vi "Simple TCP Test.vi"() -> ()   [LabVIEW 2020, in "VectoScratch.lvlib"]
uses:
  VectoScratch.lvlib
  Vecto/Connection State.ctl
  Vecto/proto/TcpClientHello/Data.ctl
  Simple TCP Handler/Simple TCP Handler.lvclass
  C:/dev/lv 2020/lv-vecto/Vecto/TCPConnectionHandler/TCPConnectionHandler.lvclass
  C:/dev/lv 2020/lv-vecto/Vecto/TCPMessageHandler/TCPMessageHandler.lvclass
  Vecto/TCPMessaging/TCPMessaging.lvclass
  Vecto/TCPMessageService/TCPMessageAPI.lvclass
  Vecto/proto/TcpClientHello/TcpClientHello.lvlib
  Vecto/Vecto.lvlib
panel:
  out "Server Read":i32
  out "Client Read":i32
  out "Server Send":i32
  in  "Server Stop":bool
  in  "Client Stop":bool
  out "Client Send":i32
  out "Server Error":errorcluster
  out "Client Error":errorcluster
  out "Server State":T1=enum."Disconnected"
  out "Client State":T1=enum."Disconnected"
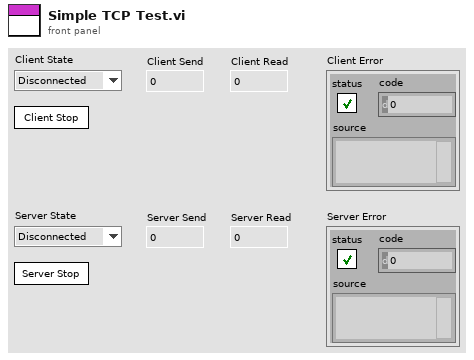
[diagram p1: front panel]
types:
  T1 = typedef "Vecto.lvlib/Connection State.ctl" = enum16{"Connected", "Disconnected"}
  T2 = typedef "TcpClientHello.lvlib/Data.ctl" = cluster{"node_id":u32, "system":string, "cluster":string, "node_name":string, "app_version":string, "config_version":string}
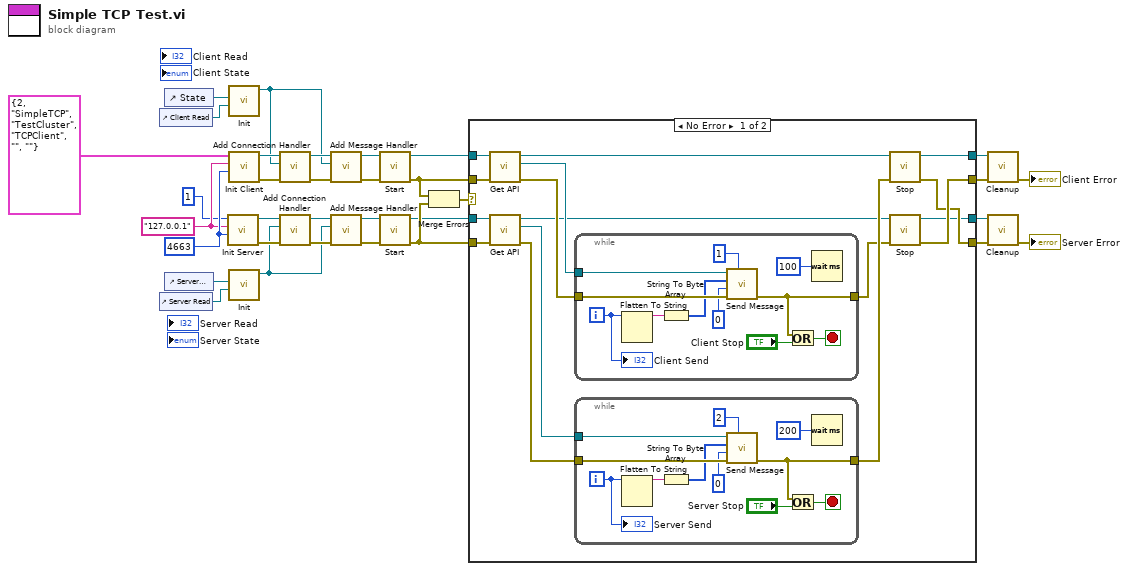
[diagram p0: block diagram]
diagram:
  w33 = u16 4663 ("Bind Port")
  w32 = "127.0.0.1" ("Bind Address")
  n1 = control-ref of="Client Read"() -> (w3:refnum<vi>)
  n2 = control-ref of="Server Read"() -> (w4:refnum<vi>)
  n3 = control-ref of="State"() -> (w30:refnum<vi>)
  n4 = control-ref of="Server State"() -> (w22:refnum<vi>)
  n5 = call "Init Server.vi"("Bind Port"=w33, "Bind Address"=w32, "Node ID"=u32 1) -> ("error out"=w16:errorcluster, "TCPMessaging out"=w17:refnum<class "TCPMessaging.lvclass">)  [unwired: 7 in]
  n6 = call "Init.vi"("Value"=w3, "State"=w30) -> ("Simple TCP Handler out"=w26:refnum<class "Simple TCP Handler.lvclass">)  [unwired: 8 in, 1 out]
  n7 = call "Init Client.vi"("Remote Port"=w33, "Remote Address"=w32, "Client Info"=T2 {"node_id"=2, "system"="SimpleTCP", "cluster"="TestCluster", "node_name"="TCPClient", "app_version"="", "config_version"=""}) -> ("error out"=w28:errorcluster, "TCPMessaging out"=w29:refnum<class "TCPMessaging.lvclass">)  [unwired: 7 in]
  n8 = call "Init.vi"("Value"=w4, "State"=w22) -> ("Simple TCP Handler out"=w2:refnum<class "Simple TCP Handler.lvclass">)  [unwired: 8 in, 1 out]
  n9 = call "Add Connection Handler.vi"("error in (no error)"=w28, "TCPConnectionHandler"=w26, "TCPMessaging in"=w29) -> ("error out"=w25:errorcluster, "TCPMessaging out"=w27:refnum<class "TCPMessaging.lvclass">)  [unwired: 7 in]
  n10 = call "Add Connection Handler.vi"("error in (no error)"=w16, "TCPConnectionHandler"=w2, "TCPMessaging in"=w17) -> ("error out"=w19:errorcluster, "TCPMessaging out"=w18:refnum<class "TCPMessaging.lvclass">)  [unwired: 7 in]
  n11 = call "Add Message Handler.vi"("error in (no error)"=w25, "TCPMessageHandler"=w26, "TCPMessaging in"=w27) -> ("error out"=w23:errorcluster, "TCPMessaging out"=w24:refnum<class "TCPMessaging.lvclass">)  [unwired: 7 in]
  n12 = call "Add Message Handler.vi"("error in (no error)"=w19, "TCPMessageHandler"=w2, "TCPMessaging in"=w18) -> ("error out"=w21:errorcluster, "TCPMessaging out"=w20:refnum<class "TCPMessaging.lvclass">)  [unwired: 7 in]
  n13 = call "Start.vi"("error in (no error)"=w23, "TCPMessaging in"=w24) -> ("error out"=w14:errorcluster, "TCPMessaging out"=w11:refnum<class "TCPMessaging.lvclass">)  [unwired: 8 in]
  n14 = call "Start.vi"("error in (no error)"=w21, "TCPMessaging in"=w20) -> ("error out"=w13:errorcluster, "TCPMessaging out"=w12:refnum<class "TCPMessaging.lvclass">)  [unwired: 8 in]
  n15 = Merge Errors(w14, w13) -> (w15:errorcluster)
  n16 = case shown="No Error" w15 {
    tunnel: w14 -> [w47 w75]
    tunnel: w13 -> [w45 w74]
    tunnel: w12 -> [w46 w73]
    tunnel: w11 -> [w48 w72]
    tunnel: [w39 w75] -> w9
    tunnel: [w37 w74] -> w7
    tunnel: [w36 w73] -> w8
    tunnel: [w38 w72] -> w10
    frame No Error {
      n17 = call "Get API.vi"("error in (no error)"=w47, "TCPMessaging in"=w48) -> ("error out"=w43:errorcluster, "TCP Service API"=w44:refnum<class "TCPMessageAPI.lvclass">, "TCPMessaging out"=w40:refnum<class "TCPMessaging.lvclass">)  [unwired: 7 in]
      n18 = call "Get API.vi"("error in (no error)"=w45, "TCPMessaging in"=w46) -> ("error out"=w34:errorcluster, "TCP Service API"=w35:refnum<class "TCPMessageAPI.lvclass">, "TCPMessaging out"=w42:refnum<class "TCPMessaging.lvclass">)  [unwired: 7 in]
      n19 = while {
        tunnel: w44 -> [w71]
        tunnel: w43 -> [w69]
        tunnel: [w61] -> w41
        i -> [w65]
        stop <- w62 stop-if-true
        n20 = Flatten To String(anything=w65) -> (data string=w67:string)  [unwired: 3 in, 2 out]
        n21 = String To Byte Array(string=w67) -> (unsigned byte array=w66:u8[])
        n22 = call "Send Message.vi"("Target Node"=u32 1, "error in (no error)"=w69, "Type ID"=u32 0, "Payload"=w66, "TCPMessageService in"=w71) -> ("error out"=w61:errorcluster)  [unwired: 5 in, 1 out]
        n23 = Or(x=w61, y="Client Stop") -> (x .or. y?=w62:bool)
        n24 = Wait (ms)(milliseconds to wait=u32 100) -> ()  [unwired: 1 out]
        "Client Send" <- w65
      }
      n25 = while {
        tunnel: w35 -> [w60]
        tunnel: w34 -> [w58]
        tunnel: [w50] -> w49
        i -> [w54]
        stop <- w51 stop-if-true
        n26 = Flatten To String(anything=w54) -> (data string=w56:string)  [unwired: 3 in, 2 out]
        n27 = String To Byte Array(string=w56) -> (unsigned byte array=w55:u8[])
        n28 = call "Send Message.vi"("Target Node"=u32 2, "error in (no error)"=w58, "Type ID"=u32 0, "Payload"=w55, "TCPMessageService in"=w60) -> ("error out"=w50:errorcluster)  [unwired: 5 in, 1 out]
        n29 = Or(x=w50, y="Server Stop") -> (x .or. y?=w51:bool)
        n30 = Wait (ms)(milliseconds to wait=u32 200) -> ()  [unwired: 1 out]
        "Server Send" <- w54
      }
      n31 = call "Stop.vi"("error in (no error)"=w49, "TCPMessaging in"=w40) -> ("error out"=w37:errorcluster, "TCPMessaging out"=w38:refnum<class "TCPMessaging.lvclass">)  [unwired: 8 in]
      n32 = call "Stop.vi"("error in (no error)"=w41, "TCPMessaging in"=w42) -> ("error out"=w39:errorcluster, "TCPMessaging out"=w36:refnum<class "TCPMessaging.lvclass">)  [unwired: 8 in]
    }
    frame Error {
    }
  }
  n33 = call "Cleanup.vi"("error in (no error)"=w9, "TCPMessaging in"=w10) -> ("error out"=→"Client Error":errorcluster)  [unwired: 9 in]
  n34 = call "Cleanup.vi"("error in (no error)"=w7, "TCPMessaging in"=w8) -> ("error out"=→"Server Error":errorcluster)  [unwired: 9 in]
